vi "ConfigureDlg.vi"(8 "error in (no error)":errorcluster, 11 "NiPxi6682 in":refnum<class "NiPxi6683H.lvclass">) -> (0 "error out":errorcluster, 2 "Changed?":bool, 3 "NiPxi6682 out":refnum<class "NiPxi6683H.lvclass">)   [LabVIEW 2014, in "SyncPlugins.lvlib" / "NiPxi6683H.lvclass"]
uses:
  NiPxi6683H.lvclass
  PXI_MultiTrig/Typedefs/clTrigger.ctl
  NiPxi6682/NiPxi6682.lvclass/NiPxi6682.ctl
  NiPxi6683H.lvclass/NiPxi6683H.ctl
  <userlib>/NIST/BaseClasses/BasePlugin_class/BasePlugin.lvclass/BasePlugin.ctl
  NiPxi6682/Accessors/Write 1PPS.vi
  NiPxi6682/Accessors/Write PgmPPS.vi
  NiPxi6682/Accessors/Write PgmPPSFreq.vi
  <userlib>/NIST/BaseClasses/BasePlugin_class/Accessors/Read PluginIniFilePath.vi
  Accessors/Write Triggers.vi
  NiPxi6682/Accessors/Read 1PPS.vi
  NiPxi6682/Accessors/Read PgmPPS.vi
  NiPxi6682/Accessors/Read PgmPPSFreq.vi
  Accessors/Read Triggers.vi
  <vilib>/Utility/config.llb/NI_LVConfig.lvlib
  PXI_MultiTrig/PXI_MultiTrig.lvclass
panel:
  in  "Triggers":T1[](array[typedef]) {"Invert?" items=["Don't Invert Signal", "Invert Signal"]; "Edge" items=["Rising Edge", "Falling Edge"]}
  in  "btnCancel":bool
  in  "btnDone":bool
  in  "Programmable Out Port":string
  in  "PgmPPSFreq":dbl=100.0 caption="Programable Out Freq"
  in  "PPS Out Port":string
  in  "Clock Card Handle":string
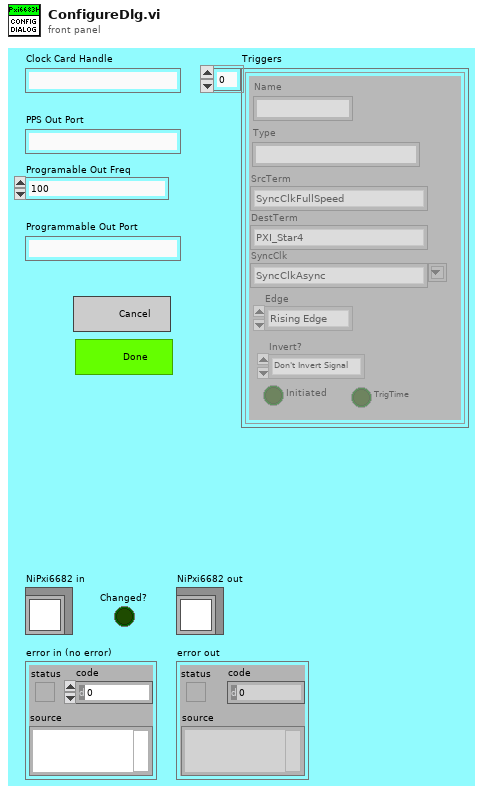
[diagram p1: front panel]
types:
  T1 = typedef "SyncPlugins.lvlib/PXI_MultiTrig.lvclass/clTrigger.ctl" = cluster{"Name":string, "DestTerm":string, "SrcTerm":string, "SyncClk":string, "Edge":i32, "Invert?":i32, "Initiated":bool, "Type":string, "TrigTime":bool}
  T2 = enum32{"Invalid", "Default", "Floating", "Floating/Auto-Hide", "Modal"}
  T3 = typedef "NI_LVConfig.lvlib/Config Data RefNum.ctl" = refnum<k1>
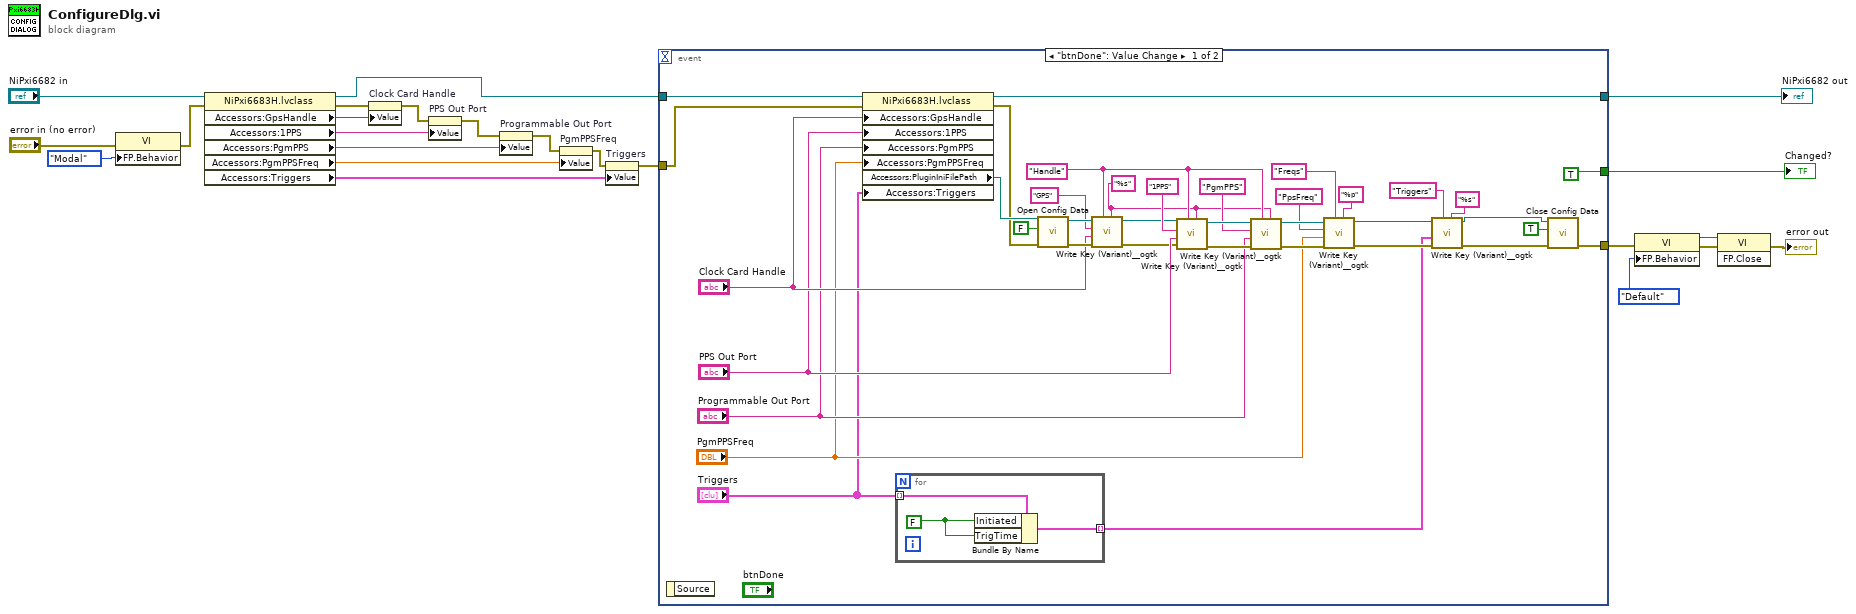
[diagram p0: block diagram]
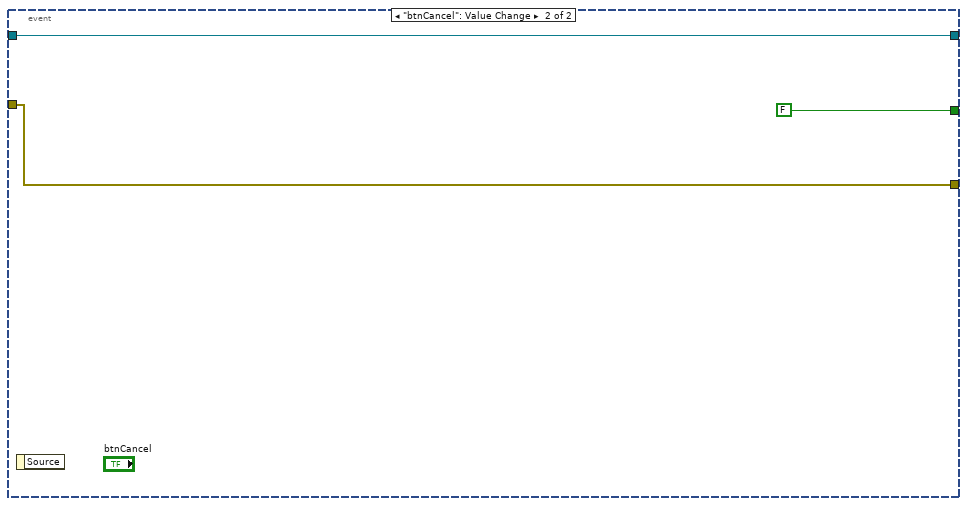
[diagram p2: hidden frame]
diagram:
  n1 = property class="VI"(error in="error in (no error)", "FP.Behavior"=T2."Modal" ("Front Panel Window:Behavior")) -> (error out=w20:errorcluster)  [unwired: 1 in, 1 out]
  n2 = property class="NiPxi6683H.lvclass"(reference="NiPxi6682 in", error in=w20) -> (reference out=w8:refnum<class "NiPxi6683H.lvclass">, error out=w15:errorcluster, "Accessors:GpsHandle"=w14:refnum<k15>, "Accessors:1PPS"=w13:tag, "Accessors:PgmPPS"=w11:tag, "Accessors:PgmPPSFreq"=w10:dbl, "Accessors:Triggers"=w3:T1[])
  n3 = property on="Clock Card Handle" class="Str"(error in=w15, "Value"=w14) -> (error out=w4:errorcluster)  [unwired: 1 in, 1 out]
  n4 = property on="PPS Out Port" class="Str"(error in=w4, "Value"=w13) -> (error out=w12:errorcluster)  [unwired: 1 in, 1 out]
  n5 = property on="Programmable Out Port" class="Str"(error in=w12, "Value"=w11) -> (error out=w9:errorcluster)  [unwired: 1 in, 1 out]
  n6 = property on="PgmPPSFreq" class="DigNum (strict)"(error in=w9, "Value"=w10) -> (error out=w1:errorcluster)  [unwired: 1 in, 1 out]
  n7 = property on="Triggers" class="Arr (strict)"(error in=w1, "Value"=w3) -> (error out=w2:errorcluster)  [unwired: 1 in, 1 out]
  n8 = event shown="[0] \"btnDone\": Value Change" {
    selector: _ -> [_ _]
    dyn-events: _ -> [_ _]
    timeout: _ -> [_ _]
    tunnel: w8 -> [w60 w65]
    tunnel: w2 -> [w34 w66]
    tunnel: [w37 w66] -> w7
    tunnel: [w36 w65] -> w6
    tunnel: [TRUE FALSE] -> w5
    event "btnDone": Value Change {
      w46 = "%s" ("float number format")
      w47 = "Handle"
      n9 = event-data() -> ()  [unwired: 1 in, 1 out]
      n10 = property class="NiPxi6683H.lvclass"(reference=w60, error in=w34, "Accessors:GpsHandle"="Clock Card Handle", "Accessors:1PPS"="PPS Out Port", "Accessors:PgmPPS"="Programmable Out Port", "Accessors:PgmPPSFreq"="PgmPPSFreq", "Accessors:Triggers"="Triggers") -> (reference out=w36:refnum<class "NiPxi6683H.lvclass">, error out=w58:errorcluster, "Accessors:PluginIniFilePath"=w59:path)
      n11 = for {
        tunnel: "Triggers" -> [w63] mode=indexing
        tunnel: [w61] -> w24 mode=indexing
        w62 = FALSE ("Initiated")
        n12 = Bundle By Name(cluster=w63, "Initiated"=w62, "TrigTime"=w62) -> (w61:T1)
      }
      n13 = call <vilib>:"Open Config Data.vi"("error in (no error)"=w58, "create file if necessary (T)"=FALSE, "configuration file path"=w59) -> ("error out"=w56:errorcluster, "refnum"=w55:T3)  [unwired: 6 in, 1 out]
      n14 = call <userlib>:"Write Key (Variant)__ogtk.vi"("float number format"=w46, "section"=w47, "error in (no error)"=w56, "key-value"="Clock Card Handle", "key (optional)"="GPS", "refnum"=w55) -> ("error out"=w32:errorcluster, "refnum out"=w33:T3)  [unwired: 4 in]
      n15 = call <userlib>:"Write Key (Variant)__ogtk.vi"("float number format"=w46, "section"=w47, "error in (no error)"=w32, "key-value"="PPS Out Port", "key (optional)"="1PPS", "refnum"=w33) -> ("error out"=w50:errorcluster, "refnum out"=w49:T3)  [unwired: 4 in]
      n16 = call <userlib>:"Write Key (Variant)__ogtk.vi"("float number format"=w46, "section"=w47, "error in (no error)"=w50, "key-value"="Programmable Out Port", "key (optional)"="PgmPPS", "refnum"=w49) -> ("error out"=w44:errorcluster, "refnum out"=w43:T3)  [unwired: 4 in]
      n17 = call <userlib>:"Write Key (Variant)__ogtk.vi"("float number format"="%p", "section"="Freqs", "error in (no error)"=w44, "key-value"="PgmPPSFreq", "key (optional)"="PpsFreq", "refnum"=w43) -> ("error out"=w31:errorcluster, "refnum out"=w30:T3)  [unwired: 4 in]
      n18 = call <userlib>:"Write Key (Variant)__ogtk.vi"("float number format"="%s", "section"="Triggers" ("float number format"), "error in (no error)"=w31, "key-value"=w24, "refnum"=w30) -> ("error out"=w26:errorcluster, "refnum out"=w27:T3)  [unwired: 5 in]
      n19 = call <vilib>:"Close Config Data.vi"("error in (no error)"=w26, "write file if changed (T)"=TRUE, "refnum"=w27) -> ("error out"=w37:errorcluster)  [unwired: 7 in, 1 out]
    }
    event "btnCancel": Value Change {
      n20 = event-data() -> ()  [unwired: 1 in, 1 out]
    }
  }
  "NiPxi6682 out" <- w6
  "Changed?" <- w5
  n21 = property class="VI"(error in=w7, "FP.Behavior"=T2."Default" ("Front Panel Window:Behavior")) -> (reference out=w19:refnum<vi>, error out=w18:errorcluster)  [unwired: 1 in]
  n22 = invoke class="VI" method="FP.Close"(reference=w19, error in=w18) -> (error out=→"error out":errorcluster)  [unwired: 1 in, 2 out]
